vi "GetProcessVariable.vi"(8 "error in":errorcluster, 10 "Channel (1-140)":u16=1 min=1 max=140 step=1, 11 "VISA resource name":refnum<visa-resource-name>) -> (0 "error out":errorcluster, 1 "Process Variable":dbl, 2 "Process Variable":string, 3 "VISA resource name out":refnum<visa-resource-name>)   [LabVIEW 2023, in "Thermotron 8800.lvlib"]
doc: "PVAR\nCommand name: Send process variable\nCommand type: Variable\nDescription: Queries the 8800 for the current process variable value of the selected channel. The channel selections are divided as follows:\nChannel Description\n1 through 4 External process variable channels \n5 through 8 Internal process variable channels\n9 - 12 Undefined \n13 - 28 Monitor channels 1 through 16\n29 - 32 Undefined \n33 - 36 System Monitor temperature channels for refrigeration system 1 (high-stage suction, high-stage discharge, low-stage suction, and low-stage discharge) \n37 - 48 System Monitor channels for refrigeration systems 2, 3, and 4 \n101 - 140 Monitor channels 1 through 40\nSyntax: PVARn?\nWhere n is the channel number (1 through 48). See Description.\nData type: Decimal\nQuery example: PVAR1?\n8800 response: -42.3 (The current channel 1 process variable value is -42.3.)"
uses:
  Thermotron 8800.lvlib
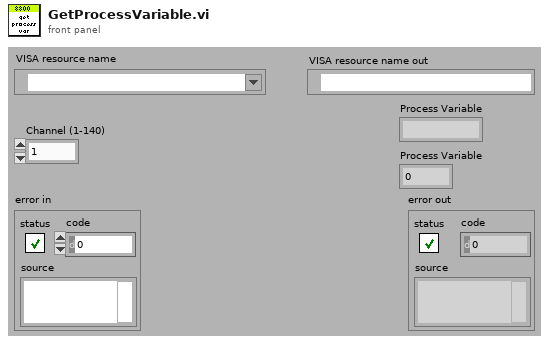
[diagram p1: front panel]
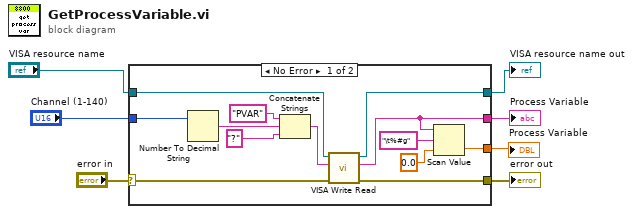
[diagram p0: block diagram]
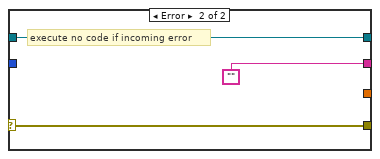
[diagram p2: hidden frame]
diagram:
  n1 = case shown="No Error" "error in" {
    selector: "error in" -> [w18 w22]
    tunnel: [w15 w22] -> w6
    tunnel: [w16 w23] -> w5
    tunnel: "VISA resource name" -> [w17 w23]
    tunnel: [w9 ""] -> w3
    tunnel: "Channel (1-140)" -> [w12 _]
    tunnel: [w8 _] -> w1
    frame No Error {
      n2 = Number To Decimal String(number=w12) -> (decimal integer string=w13:string)  [unwired: 1 in]
      n3 = Concatenate Strings("PVAR" ("8800 Command"), w13, "?" ("8800 Command")) -> (w20:string)
      n4 = call "VISA Write Read.vi"("error in (no error)"=w18, "8800 Command"=w20, "VISA Refnum in"=w17) -> ("error out"=w15:errorcluster, "read buffer"=w9:string, "VISA Refnum out"=w16:refnum<visa-resource-name>)  [unwired: 6 in]
      n5 = Scan Value(string=w9, format string="\t%#g", default (0 dbl)=0.0) -> (value=w8:dbl)  [unwired: 1 out]
    }
    frame Error {
      # "execute no code if incoming error"
    }
  }
  "VISA resource name out" <- w5
  "error out" <- w6
  "Process Variable" <- w3
  "Process Variable" <- w1
